vi "Open-DOTNET.vi"(8 "error in (no error)":errorcluster, 11 "SM1000-control in":T1) -> (0 "error out":errorcluster, 1 "Succes?":bool, 3 "SM1000-control out":T1)   [LabVIEW 2013, in "SLMControl.lvlib" / "SM1000.lvclass"]
uses:
  SM1000.lvclass
  Object-reference.ctl
  C:/Users/vangeste/Desktop/2015-06-02 - SLM - MAIF/HC-HardwareCharacterization/Sources/SM1000/LECBroadcast.dll
  HC-HardwareCharacterization/Sources/SM1000/LECBroadcast.dll
  C:/Users/vangeste/Desktop/2015-06-02 - SLM - MAIF/HC-HardwareCharacterization/Sources/SM1000/LECSession.dll
  HC-HardwareCharacterization/Sources/SM1000/LECSession.dll
  SM1000.lvclass/SM1000.ctl
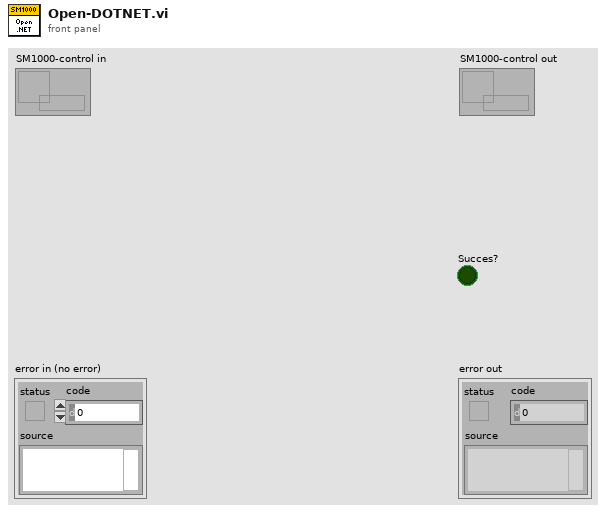
[diagram p1: front panel]
types:
  T1 = typedef "SLMControl.lvlib/SM1000.lvclass/Object-reference.ctl" = refnum<data-value>
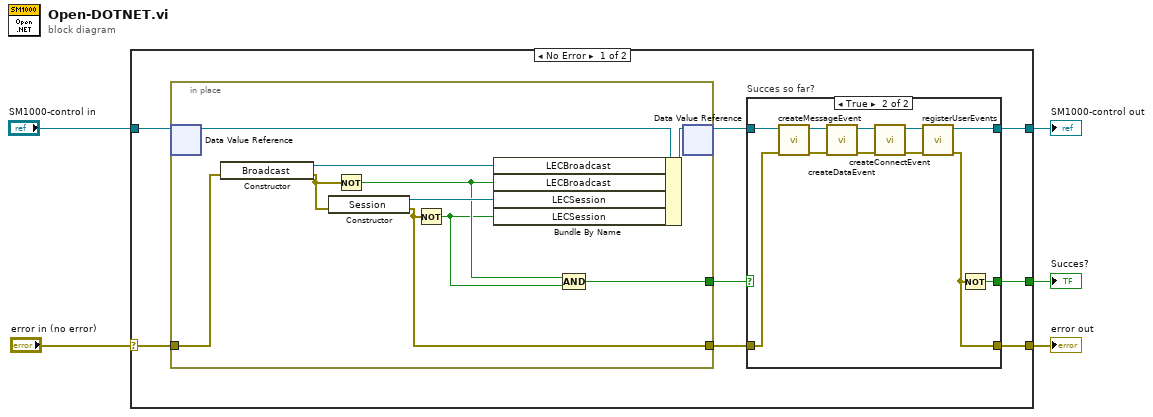
[diagram p0: block diagram]
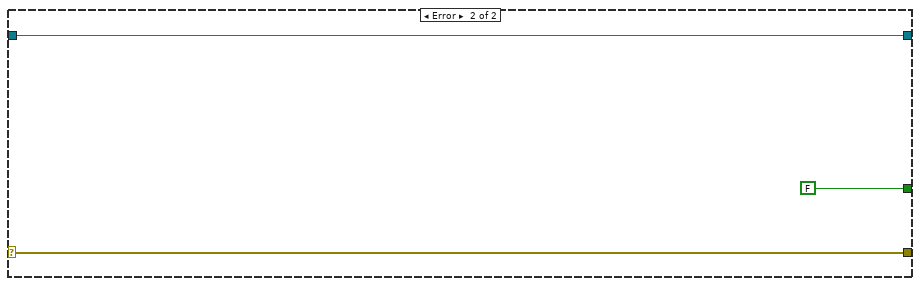
[diagram p3: hidden frame]
diagram:
  n1 = case shown="No Error" "error in (no error)" {
    selector: "error in (no error)" -> [w13 w40]
    tunnel: [w9 w40] -> w4
    tunnel: [w10 w39] -> w2
    tunnel: "SM1000-control in" -> [w12 w39]
    tunnel: [w6 FALSE] -> w1
    frame No Error {
      n2 = in-place {
        in-place-border: w13 -> [w35]
        in-place-border: [w31] -> w8
        in-place-border: [w28] -> w7
        n3 = in-place-dvr #1(w12) -> (w37:refnum<class "SM1000.lvclass">)  [unwired: 1 out]
        n4 = constructor class="Broadcast"(error in=w35) -> (reference out=w34:refnum<k24>, error out=w33:errorcluster)  [unwired: 2 in, 1 out]
        n5 = constructor class="Session"(error in=w33) -> (reference out=w32:refnum<k24>, error out=w31:errorcluster)  [unwired: 2 in, 1 out]
        n6 = Not(x=w33) -> (.not. x?=w30:bool)
        n7 = Not(x=w31) -> (.not. x?=w29:bool)
        n8 = Bundle By Name(cluster=w37, "LECBroadcast"=w34, "LECBroadcast"=w30, "LECSession"=w32, "LECSession"=w29) -> (w36:refnum<class "SM1000.lvclass">)
        n9 = Compound Arithmetic op=AND(w30, w29) -> (w28:bool)
        n10 = in-place-dvr #1(w36) -> (w11:T1)  [unwired: 1 out]
      }
      n11 = case "Succes so far?" shown="True" w7 {
        selector: w7 -> [w15 _]
        tunnel: w11 -> [w16 w17]
        tunnel: [w16 w25] -> w10
        tunnel: [w14 w23] -> w9
        tunnel: w8 -> [w14 w18]
        tunnel: [w15 w24] -> w6
        frame False {
        }
        frame True {
          n12 = call "createMessageEvent.vi"("error in (no error)"=w18, "SM1000-control in"=w17) -> ("error out"=w27:errorcluster, "SM1000-control out"=w26:T1)  [unwired: 7 in, 1 out]
          n13 = call "createDataEvent.vi"("error in (no error)"=w27, "SM1000-control in"=w26) -> ("error out"=w19:errorcluster, "SM1000-control out"=w22:T1)  [unwired: 7 in, 1 out]
          n14 = call "createConnectEvent.vi"("error in (no error)"=w19, "SM1000-control in"=w22) -> ("error out"=w20:errorcluster, "SM1000-control out"=w21:T1)  [unwired: 7 in, 1 out]
          n15 = call "registerUserEvents.vi"("error in (no error)"=w20, "SM1000-control in"=w21) -> ("error out"=w23:errorcluster, "SM1000-control out"=w25:T1)  [unwired: 7 in, 1 out]
          n16 = Not(x=w23) -> (.not. x?=w24:bool)
        }
      }
    }
    frame Error {
    }
  }
  "error out" <- w4
  "SM1000-control out" <- w2
  "Succes?" <- w1
